vi "Write Loop.vi"(8 "error in (no error)":errorcluster, 11 "WAMP Client in":refnum<class "WAMP Client.lvclass">) -> (0 "error out":errorcluster, 3 "WAMP Client out":refnum<class "WAMP Client.lvclass">)   [LabVIEW 2020, in "wamplv.lvlib" / "WAMP Client.lvclass"]
uses:
  WAMP Client.lvclass
  WAMP Client.lvclass/WAMP Client.ctl
  TypeDef/Termination Reason Enum.ctl
  Private/Comm Handlers/ICommHandler/ICommHandler.lvclass
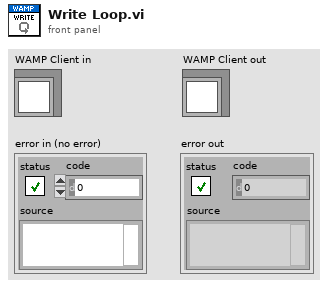
[diagram p1: front panel]
types:
  T1 = typedef "wamplv.lvlib/WAMP Client.lvclass/Termination Reason Enum.ctl" = enum16{"Goodbye Received", "Abort Received", "Send Goodbye", "Send Abort", "Read Loop Failure", "Write Loop Failure", "Message Loop Failure"}
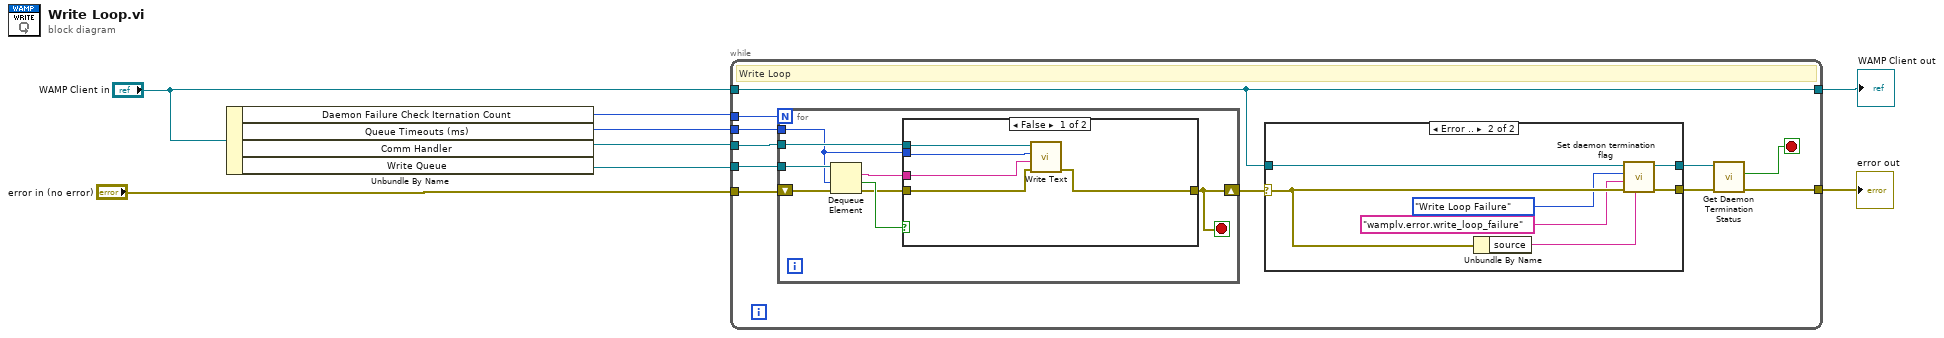
[diagram p0: block diagram]
diagram:
  n1 = Unbundle By Name("WAMP Client in") -> ("Daemon Failure Check Iternation Count"=w2:i32, "Queue Timeouts (ms)"=w3:i32, "Comm Handler"=w8:refnum<class "ICommHandler.lvclass">, "Write Queue"=w7:refnum<queue>)
  n2 = while {
    tunnel: w7 -> [w19]
    tunnel: w8 -> [w18]
    tunnel: "error in (no error)" -> [w17]
    tunnel: [w12] -> w5
    tunnel: "WAMP Client in" -> [w9]
    tunnel: w3 -> [w10]
    tunnel: w2 -> [w11]
    tunnel: [w9] -> w1
    stop <- w13 stop-if-true
    # "Write Loop"
    n3 = for {
      N: w11 -> [_]
      tunnel: w19 -> [w27]
      tunnel: w18 -> [w26]
      shift-right: [w21] -> w16
      shift-left: w17 -> [w22]
      tunnel: w10 -> [w20]
      stop <- w21 stop-if-true
      n4 = Dequeue Element(queue=w27, timeout in ms (-1)=w20, error in (no error)=w22) -> (element=w25:string, timed out?=w24:bool, error out=w23:errorcluster)  [unwired: 1 out]
      n5 = case shown="False" w24 {
        tunnel: w26 -> [w32 _]
        tunnel: w25 -> [w29 _]
        tunnel: w23 -> [w31 w33]
        tunnel: [w30 w33] -> w21
        tunnel: w20 -> [w28 _]
        frame False {
          n6 = call-dynamic "Write Text.vi"("error in (no error)"=w31, "String"=w29, "timeout ms (5000)"=w28, "ICommHandler in"=w32) -> ("error out"=w30:errorcluster)  [unwired: 6 in, 1 out]
        }
        frame True {
          # "Queue is empty, do nothing"
        }
      }
    }
    n7 = case shown="Error .." w16 {
      selector: w16 -> [w35 w41]
      tunnel: [w35 w42] -> w15
      tunnel: [w34 w40] -> w14
      tunnel: w9 -> [w34 w36]
      frame No Error {
      }
      frame Error {
        n8 = Unbundle By Name(w41) -> ("source"=w37:string)
        n9 = call "Set daemon termination flag.vi"("Message"=w37, "error in (no error)"=w41, "Reason URI"="wamplv.error.write_loop_failure" ("Error URI"), "Reason"=Termination_Reason_Enum."Write Loop Failure" ("Termination Reason"), "WAMP Client (in)"=w36) -> ("error out"=w42:errorcluster, "WAMP Client (out)"=w40:refnum<class "WAMP Client.lvclass">)  [unwired: 5 in]
      }
    }
    n10 = call "Get Daemon Termination Status.vi"("error in (no error)"=w15, "WAMP Client in"=w14) -> ("error out"=w12:errorcluster, "Terminate?"=w13:bool)  [unwired: 6 in, 2 out]
  }
  "error out" <- w5
  "WAMP Client out" <- w1
